vi "Write Player Info.vi"(8 "error in (no error)":errorcluster, 10 "Player Info":T1={"Name"="", "Color Box"=0, "Gloat Phrase"="All your base are belong to us!!"}, 11 "Runner in":refnum<class "Runner.lvclass">) -> (0 "error out":errorcluster, 3 "Runner out":refnum<class "Runner.lvclass">)   [LabVIEW 2014, in "Runner.lvclass"]
uses:
  Runner.lvclass
  Player Info.ctl
  SquareBattle.lvclass
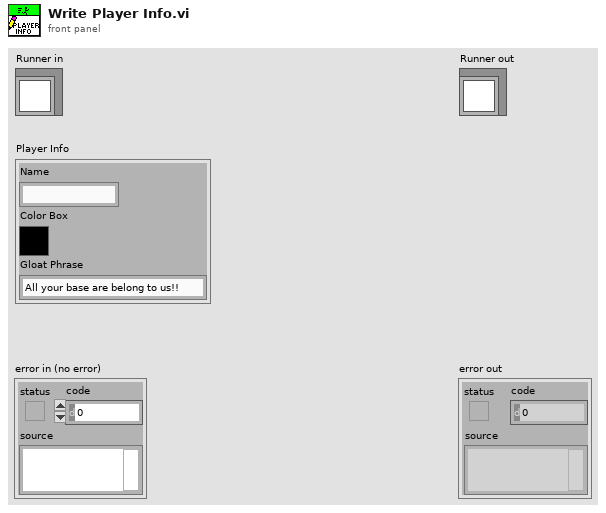
[diagram p1: front panel]
types:
  T1 = typedef "SquareBattle.lvclass/Player Info.ctl" = cluster{"Name":string, "Color Box":u32, "Gloat Phrase":string}
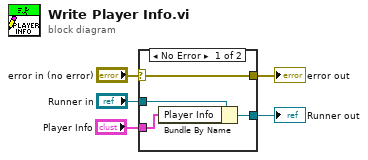
[diagram p0: block diagram]
diagram:
  n1 = case shown="No Error" "error in (no error)" {
    selector: "error in (no error)" -> [w9 w10]
    tunnel: [w9 w10] -> w4
    tunnel: [w7 w11] -> w2
    tunnel: "Runner in" -> [w8 w11]
    tunnel: "Player Info" -> [w6 _]
    frame No Error {
      n2 = Bundle By Name(cluster=w8, "Player Info"=w6) -> (w7:refnum<class "Runner.lvclass">)
    }
    frame Error {
    }
  }
  "error out" <- w4
  "Runner out" <- w2
